vi "Write XY.vi"(5 "Tag.lvclass":refnum<class "Tag.lvclass">, 7 "TagX":dbl, 9 "TagY":dbl, 12 "error in (no error)":errorcluster) -> (8 "Tag Out":refnum<class "Tag.lvclass">, 14 "error out":errorcluster)   [LabVIEW 2014, in "Tag.lvclass"]
uses:
  Tag.lvclass
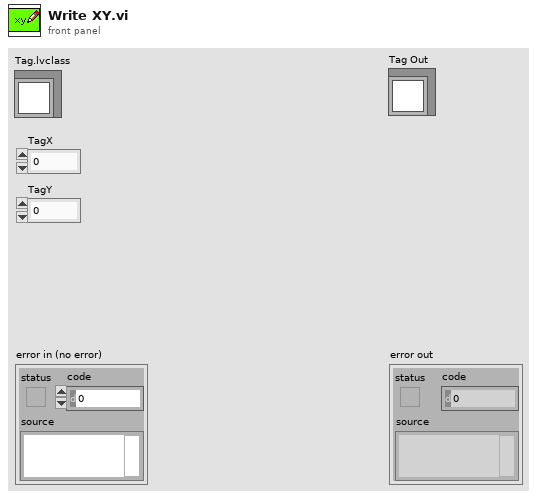
[diagram p1: front panel]
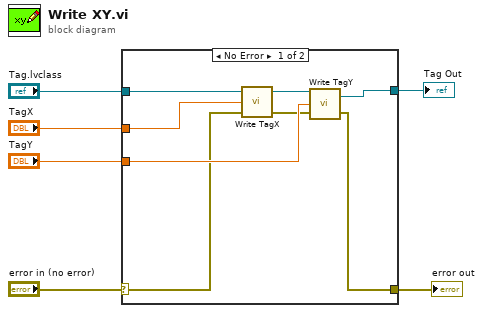
[diagram p0: block diagram]
diagram:
  n1 = case shown="No Error" "error in (no error)" {
    selector: "error in (no error)" -> [w9 w16]
    tunnel: [w7 w16] -> w5
    tunnel: "Tag.lvclass" -> [w10 w15]
    tunnel: [w11 w15] -> w3
    tunnel: "TagY" -> [w12 _]
    tunnel: "TagX" -> [w13 _]
    frame No Error {
      n2 = call-dynamic "Write TagX.vi"("error in (no error)"=w9, "TagX"=w13, "Tag in"=w10) -> ("error out"=w8:errorcluster, "Tag out"=w14:refnum<class "Tag.lvclass">)  [unwired: 1 in]
      n3 = call-dynamic "Write TagY.vi"("error in (no error)"=w8, "TagY"=w12, "Tag in"=w14) -> ("error out"=w7:errorcluster, "Tag out"=w11:refnum<class "Tag.lvclass">)
    }
    frame Error {
    }
  }
  "error out" <- w5
  "Tag Out" <- w3
